vi "CS_MFA_Coms_and_Status_Check.vi"(11 "VISA resource name":refnum<visa-resource-name>) -> (1 "Temperature":sgl, 2 "DriveRatedCurrent":sgl, 3 "AAABuild":i32)   [LabVIEW 2018]
uses:
  <vilib>/Instr/_visa.llb/VISA Configure Serial Port (Instr).vi
panel:
  out "error Temperature":errorcluster
  out "error DriveRatedCurrent":errorcluster
  out "error AAABuild":errorcluster
  out "error MicroFlexLink":errorcluster
  in  "MintController":refnum<k7>(container)
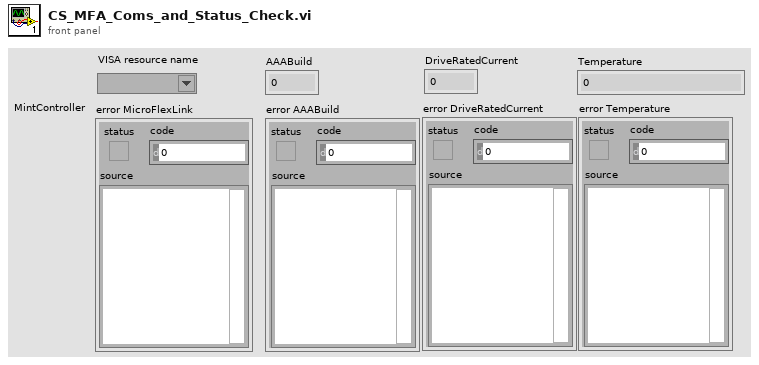
[diagram p1: front panel]
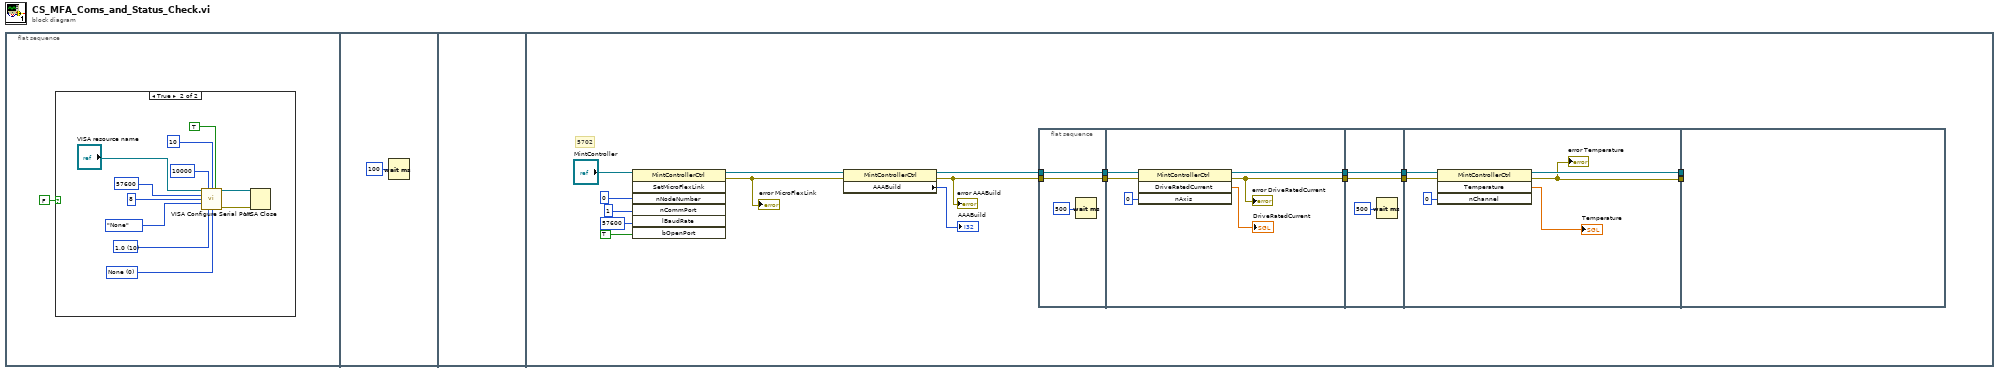
[diagram p0: block diagram]
diagram:
  n1 = flat-sequence {
    frame #0 {
      n2 = case shown="True" FALSE {
        frame False {
        }
        frame True {
          w10 = u16 0 items=["None", "XON/XOFF", "RTS/CTS", "XON/XOFF & RTS/CTS", "DTR/DSR", "XON/XOFF & DTR/DSR"] ("flow control (0:none)")
          w11 = u16 10 items=["1.0"=10, "1.5"=15, "2.0"=20] ("stop bits (10: 1 bit)")
          n3 = call-poly "VISA Configure Serial Port"("VISA resource name"="VISA resource name", "timeout (10sec)"=u32 10000, "termination char\n(0xA = '\\n' = LF)"=u8 10 ("termination char\n(0xA = '\\n' = LF)"), "Enable Termination\nChar (T)"=TRUE ("Enable Termination\nChar (T)"), "baud rate (9600)"=u32 57600, "data bits (8)"=u16 8, "parity (0:none)"=enum16{"None", "Odd", "Even", "Mark", "Space"}."None", "stop bits (10: 1 bit)"=w11, "flow control (0:none)"=w10) -> ("VISA resource name out"=w3:refnum<visa-resource-name>, "error out"=w2:errorcluster)  [unwired: 5 in]
          n4 = VISA Close(VISA resource name=w3, error in (no error)=w2) -> ()  [unwired: 1 out]
        }
      }
    }
    frame #1 {
      n5 = Wait (ms)(milliseconds to wait=u32 100) -> ()  [unwired: 1 out]
    }
    frame #2 {
    }
    frame #3 {
      # "5702"
      n6 = invoke class="MintControllerCtrl" method="SetMicroFlexLink"(reference="MintController", "nNodeNumber"=i16 0 ("nNode"), "nCommPort"=i16 1, "lBaudRate"=57600, "bOpenPort"=TRUE) -> (reference out=w20:refnum<k7>, error out=w18:errorcluster)  [unwired: 2 in, 5 out]
      "error MicroFlexLink" <- w18
      n7 = property class="MintControllerCtrl"(reference=w20, error in=w18) -> (reference out=w17:refnum<k7>, error out=w16:errorcluster, "AAABuild"=→"AAABuild":i32)
      "error AAABuild" <- w16
      n8 = flat-sequence {
        tunnel: w16 -> [w33]
        tunnel: w17 -> [w34]
        tunnel: [w34] -> w31
        tunnel: [w33] -> w30
        tunnel: [w36] -> w29
        tunnel: [w35] -> w28
        tunnel: w31 -> [w40]
        tunnel: w30 -> [w39]
        tunnel: w29 -> [w43]
        tunnel: [w43] -> w27
        tunnel: w28 -> [w42]
        tunnel: [w42] -> w26
        tunnel: w27 -> [w47]
        tunnel: w26 -> [w46]
        tunnel: [w45] -> w15
        tunnel: [w44] -> w14
        tunnel: w15 -> [_]
        tunnel: w14 -> [_]
        frame #0 {
          n9 = Wait (ms)(milliseconds to wait=u32 500) -> ()  [unwired: 1 out]
        }
        frame #1 {
          n10 = invoke class="MintControllerCtrl" method="DriveRatedCurrent"(reference=w40, error in=w39, "nAxis"=i16 0) -> (reference out=w35:refnum<k7>, error out=w36:errorcluster, "DriveRatedCurrent"=→"DriveRatedCurrent":sgl)  [unwired: 1 in, 1 out]
          "error DriveRatedCurrent" <- w36
        }
        frame #2 {
          n11 = Wait (ms)(milliseconds to wait=u32 500) -> ()  [unwired: 1 out]
        }
        frame #3 {
          n12 = invoke class="MintControllerCtrl" method="Temperature"(reference=w46, error in=w47, "nChannel"=i16 0) -> (reference out=w45:refnum<k7>, error out=w44:errorcluster, "Temperature"=→"Temperature":sgl)  [unwired: 1 in, 1 out]
          "error Temperature" <- w44
        }
        frame #4 {
        }
      }
    }
  }
